vi "PH_Cont-601k_PSU.ProcCases.vi"(0 "i ref in":refnum<vi>, 1 "selector":string, 2 "Data":T1, 3 "call cluster":T2={"Object"="", "Selector"="", "CallType"=enum."synchronous", "Async Object"="", "Async Selector"="", "Data Descriptor"="", "Data"=[], "Error #"=0, "Expire"=0}, 5 "error in (no error)":errorcluster) -> (14 "i ref out":refnum<vi>, 17 "answer cluster":T2={"Object"="", "Selector"="", "CallType"=enum."synchronous", "Async Object"="", "Async Selector"="", "Data Descriptor"="", "Data"=[], "Error #"=0, "Expire"=0}, 19 "error out":errorcluster)   [LabVIEW 2014, in "PH_Cont-601k_PSU.lvlib"]
doc: "This method is called by a process from within the default case in the event loop. The methods of a class that are linked to events will be called from THIS method. Add your code here."
uses:
  PH_Cont-601k_PSU.lvlib
  CS_Core/CSSystem/CoreDefs/CoreDefs.call_type.ctl
  CS_Core/BaseProcess/BaseProcess.descriptor string definition.ctl
  CS_Core/CSSystem/CoreDefs/CoreDefs.rawDataType.ctl
  PH_Cont-601k_PSU.Readyness Device.ctl
  PH_Cont-601k_PSU.Readyness Program.ctl
  CS_Core/CSSystem/CoreLib/CoreLib.string 2 byte array.vi
  CS_Core/CSSystem/CoreLib/CoreLib.byte array 2 int.vi
  CS_Core/CSSystem/CoreLib/CoreLib.byte array 2 short.vi
  CS_Core/CSSystem/CoreLib/CoreLib.byte array 2 double.vi
  CS_Core/BaseProcess/BaseProcess.lvlib
  CS_Core/CSSystem/CoreLib/CoreLib.lvlib
  CS_Core/CAEObj/CAEObj.lvlib
  PH_Basics/PH_Common/PH_Common.lvlib
  PH_Basics/PH_Class/PH_Class.lvlib
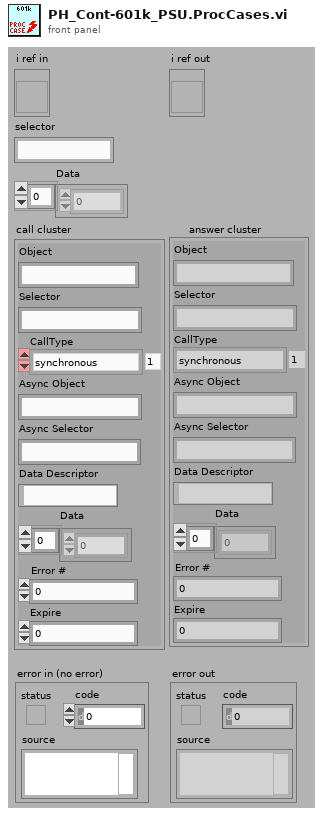
[diagram p1: front panel]
types:
  T1 = typedef "CoreDefs.rawDataType.ctl" = i8[]
  T2 = typedef "CoreDefs.call_type.ctl" = cluster{"Object":string, "Selector":string, "CallType":enum16{"simple", "synchronous", "asynchronous"}, "Async Object":string, "Async Selector":string, "Data Descriptor":T3, "Data":T1, "Error #":i32, "Expire":u32}
  T3 = typedef "BaseProcess.lvlib/BaseProcess.descriptor string definition.ctl" = string
  T4 = typedef "PH_Cont-601k_PSU.lvlib/PH_Cont-601k_PSU.Readyness Device.ctl" = enum32{"OFF", "CONNECTING", "CONNECTED", "OPERATING", "EOC", "ERROR"}
  T5 = typedef "PH_Cont-601k_PSU.lvlib/PH_Cont-601k_PSU.Readyness Program.ctl" = enum32{"OFF", "POWER", "INTERLOCK"}
  T6 = typedef "PH_Cont-601k_PSU.lvlib/PH_Cont-601k_PSU.Mode.ctl" = enum32{"STOP", "STANDBY", "READY", "EMISSION", "ERROR"}
  T7 = typedef "PH_Cont-601k_PSU.lvlib/PH_Cont-601k_PSU.i attribute.ctl" = cluster{"GUI Refs":T8, "Interlock":bool, "Service ID applied Voltage":i32, "Device Settings":cluster{"Configuration":T9, "Flash Interval [s]":dbl, "Mode":T6, "Voltage [V]":u16, "Charge":bool, "VISA resource name":refnum<visa-resource-name>}, "Readyness":T10, "Information":cluster{"VISA resource name":refnum<visa-resource-name>, "Tagname Power On":string, "Interlock":cluster{"Instance":string, "Tagname":string}, "Limits [V]":cluster{"Lower":dbl, "Upper":dbl}, "Tagname PSU On":string}, "R2S":bool, "Charge is allowed":bool}
  T8 = typedef "PH_Cont-601k_PSU.lvlib/PH_Cont-601k_PSU.GUI Refs.ctl" = cluster{"Power On":refnum<vi>, "Hard- and Software":refnum<vi>, "Device Status":refnum<vi>, "Device Error":refnum<vi>, "Configuration":refnum<vi>, "Flash Interval [s]":refnum<vi>, "Interlock":refnum<vi>, "Interlock Indicator":refnum<vi>, "Voltage [V]":refnum<vi>, "Readyness":refnum<vi>, "Mode":refnum<vi>, "Reset Error":refnum<vi>, "Expert working":refnum<vi>, "Charge":refnum<vi>, "PSU On":refnum<vi>}
  T9 = typedef "PH_Cont-601k_PSU.lvlib/PH_Cont-601k_PSU.Configuration.ctl" = u16
  T10 = typedef "PH_Cont-601k_PSU.lvlib/PH_Cont-601k_PSU.Readyness.ctl" = cluster{"Program":T5, "Device":T4}
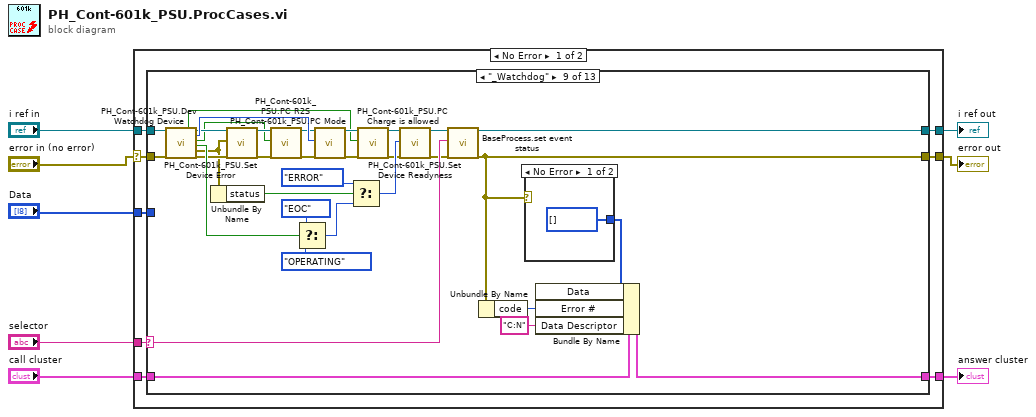
[diagram p0: block diagram]
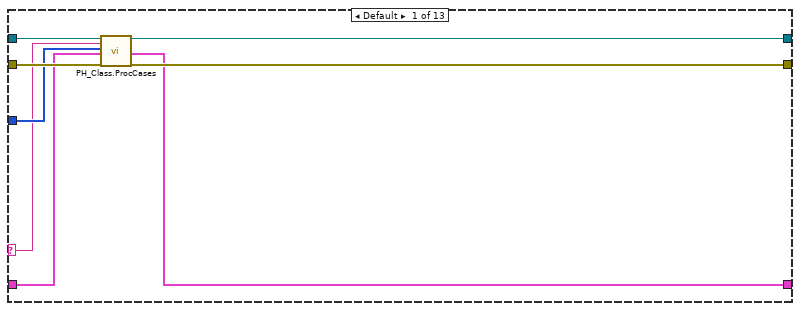
[diagram p2: hidden frame]
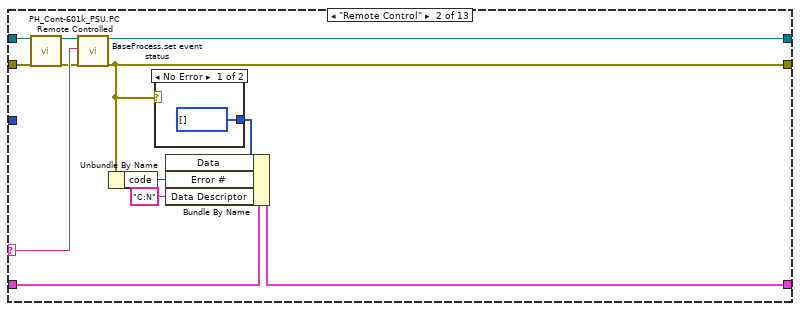
[diagram p3: hidden frame]
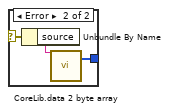
[diagram p4: hidden frame]
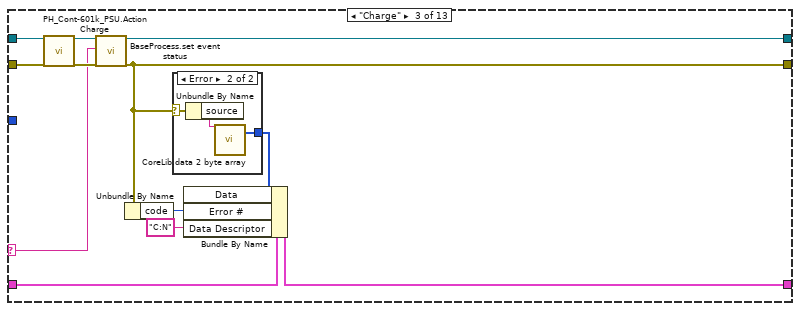
[diagram p5: hidden frame]
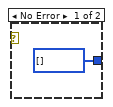
[diagram p6: hidden frame]
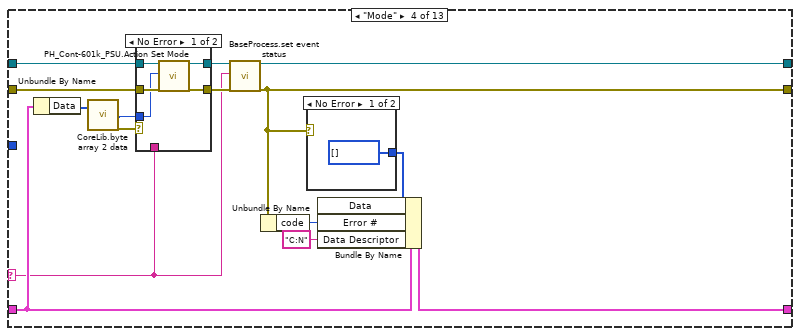
[diagram p7: hidden frame]
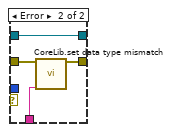
[diagram p8: hidden frame]
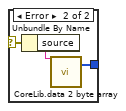
[diagram p9: hidden frame]
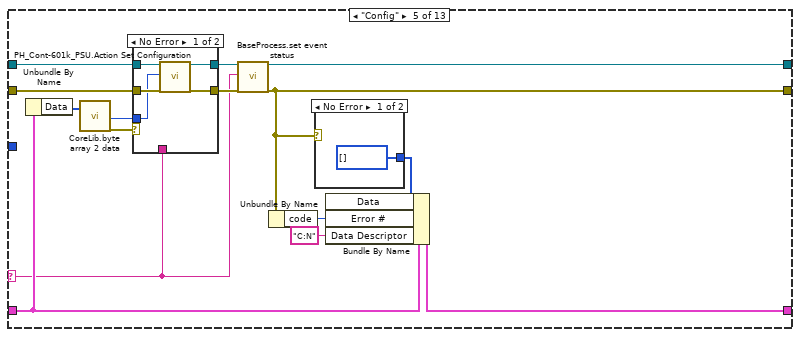
[diagram p10: hidden frame]
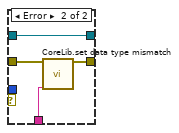
[diagram p11: hidden frame]
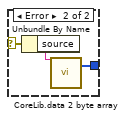
[diagram p12: hidden frame]
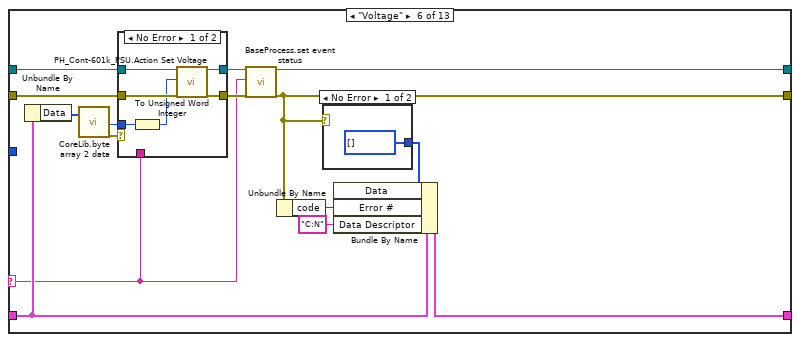
[diagram p13: hidden frame]
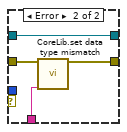
[diagram p14: hidden frame]
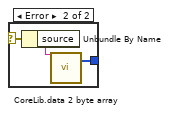
[diagram p15: hidden frame]
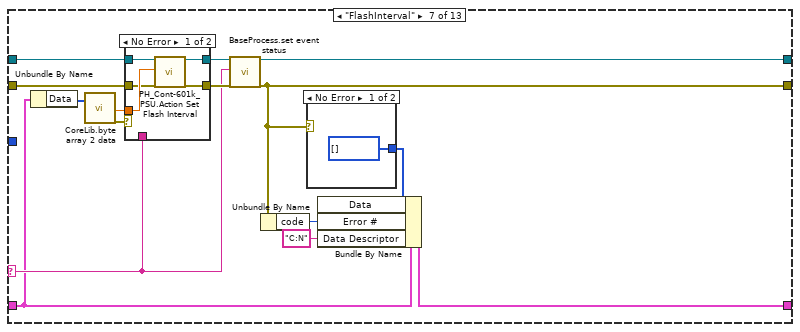
[diagram p16: hidden frame]
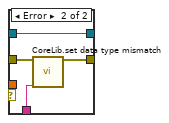
[diagram p17: hidden frame]
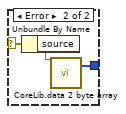
[diagram p18: hidden frame]
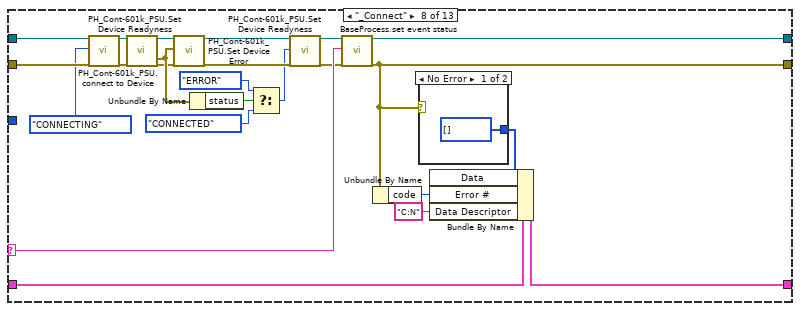
[diagram p19: hidden frame]
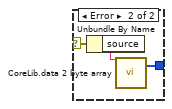
[diagram p20: hidden frame]
diagram:
  n1 = case shown="No Error" "error in (no error)" {
    selector: "error in (no error)" -> [w9 w425]
    tunnel: "selector" -> [w16 _]
    tunnel: [w15 w426] -> w7
    tunnel: "Data" -> [w14 _]
    tunnel: "call cluster" -> [w13 w426]
    tunnel: "i ref in" -> [w12 w427]
    tunnel: [w11 w427] -> w3
    tunnel: [w10 w425] -> w2
    frame No Error {
      n2 = case shown="\"_Watchdog\"" w16 {
        selector: w16 -> [w18 w32 w42 w57 w85 w113 w148 w186 w223 w240 w271 w319 w369]
        tunnel: w14 -> [w19 _ _ _ _ _ _ _ _ _ w270 w318 w368]
        tunnel: w12 -> [w17 w35 w41 w63 w91 w119 w147 w176 w211 w236 w264 w312 w362]
        tunnel: [w24 w27 w49 w68 w96 w124 w153 w190 w227 w246 w277 w325 w375] -> w11
        tunnel: w13 -> [w20 w30 w43 w60 w88 w116 w144 w187 w224 w241 w274 w322 w372]
        tunnel: [w21 w29 w50 w69 w97 w125 w154 w191 w228 w247 w280 w328 w378] -> w15
        tunnel: w9 -> [w23 w36 w46 w62 w90 w118 w146 w174 w210 w235 w275 w323 w373]
        tunnel: [w22 w26 w48 w67 w95 w123 w152 w189 w226 w245 w278 w326 w376] -> w10
        frame Default {
          n3 = call "PH_Class.ProcCases.vi"("i ref in"=w17, "selector"=w18, "Data"=w19, "call cluster"=w20, "error in (no error)"=w23) -> ("i ref out"=w24:refnum<vi>, "answer cluster"=w21:T2, "error out"=w22:errorcluster)  [unwired: 12 in]
        }
        frame "Remote Control" {
          n4 = call "PH_Cont-601k_PSU.PC Remote Controlled.vi"("i ref in"=w35, "error in (no error)"=w36) -> ("i ref out"=w31:refnum<vi>, "error out"=w28:errorcluster)  [unwired: 16 in]
          n5 = call "BaseProcess.set event status.vi"("i ref in"=w31, "EventStatus"=w32, "error in (no error)"=w28) -> ("i ref out"=w27:refnum<vi>, "error out"=w26:errorcluster)  [unwired: 14 in, 1 out]
          n6 = Unbundle By Name(w26) -> ("code"=w34:i32)
          n7 = case shown="No Error" w26 {
            selector: w26 -> [_ w40]
            tunnel: [T1 [] ("byteArray out") w39] -> w33
            frame No Error {
            }
            frame Error {
              n8 = Unbundle By Name(w40) -> ("source"=w38:string)
              n9 = call-poly "CoreLib.data 2 byte array.vi"("string"=w38) -> ("byteArray out"=w39:T1)  [unwired: 18 in]
            }
          }
          n10 = Bundle By Name(cluster=w30, "Data"=w33, "Error #"=w34, "Data Descriptor"="C:N") -> (w29:T2)
        }
        frame "Charge" {
          n11 = call "PH_Cont-601k_PSU.Action Charge.vi"("VI in"=w41, "error in (no error)"=w46) -> ("VI out"=w45:refnum<vi>, "error out"=w44:errorcluster)  [unwired: 16 in]
          n12 = call "BaseProcess.set event status.vi"("i ref in"=w45, "EventStatus"=w42, "error in (no error)"=w44) -> ("i ref out"=w49:refnum<vi>, "error out"=w48:errorcluster)  [unwired: 14 in, 1 out]
          n13 = Unbundle By Name(w48) -> ("code"=w52:i32)
          n14 = case shown="Error" w48 {
            selector: w48 -> [_ w56]
            tunnel: [T1 [] ("byteArray out") w55] -> w51
            frame No Error {
            }
            frame Error {
              n15 = Unbundle By Name(w56) -> ("source"=w54:string)
              n16 = call-poly "CoreLib.data 2 byte array.vi"("string"=w54) -> ("byteArray out"=w55:T1)  [unwired: 18 in]
            }
          }
          n17 = Bundle By Name(cluster=w43, "Data"=w51, "Error #"=w52, "Data Descriptor"="C:N") -> (w50:T2)
        }
        frame "Mode" {
          n18 = Unbundle By Name(w60) -> ("Data"=w61:T1)
          n19 = call-poly "CoreLib.byte array 2 data.vi"("byteArray"=w61) -> ("i32"=w59:i32, "error out"=w58:errorcluster)  [unwired: 16 in, 1 out]
          n20 = case shown="No Error" w58 {
            tunnel: [w76 w78] -> w65
            tunnel: [w75 w77] -> w64
            tunnel: w63 -> [w74 w77]
            tunnel: w62 -> [w73 w80]
            tunnel: w59 -> [w72 _]
            tunnel: w57 -> [_ w79]
            frame No Error {
              n21 = call "PH_Cont-601k_PSU.Action Set Mode.vi"("VI in"=w74, "Mode"=w72, "error in (no error)"=w73) -> ("VI out"=w75:refnum<vi>, "error out"=w76:errorcluster)  [unwired: 15 in]
            }
            frame Error {
              n22 = call "CoreLib.set data type mismatch.vi"("error in (no error)"=w80, "error source"=w79) -> ("error out"=w78:errorcluster)  [unwired: 17 in]
            }
          }
          n23 = call "BaseProcess.set event status.vi"("i ref in"=w64, "EventStatus"=w57, "error in (no error)"=w65) -> ("i ref out"=w68:refnum<vi>, "error out"=w67:errorcluster)  [unwired: 14 in, 1 out]
          n24 = Unbundle By Name(w67) -> ("code"=w71:i32)
          n25 = case shown="No Error" w67 {
            selector: w67 -> [_ w84]
            tunnel: [T1 [] ("byteArray out") w83] -> w70
            frame No Error {
            }
            frame Error {
              n26 = Unbundle By Name(w84) -> ("source"=w82:string)
              n27 = call-poly "CoreLib.data 2 byte array.vi"("string"=w82) -> ("byteArray out"=w83:T1)  [unwired: 18 in]
            }
          }
          n28 = Bundle By Name(cluster=w60, "Data"=w70, "Error #"=w71, "Data Descriptor"="C:N") -> (w69:T2)
        }
        frame "Config" {
          n29 = Unbundle By Name(w88) -> ("Data"=w89:T1)
          n30 = call-poly "CoreLib.byte array 2 data.vi"("byteArray"=w89) -> ("i16"=w87:i16, "error out"=w86:errorcluster)  [unwired: 16 in, 1 out]
          n31 = case shown="No Error" w86 {
            tunnel: [w104 w107] -> w93
            tunnel: [w103 w106] -> w92
            tunnel: w91 -> [w102 w106]
            tunnel: w90 -> [w101 w108]
            tunnel: w87 -> [w100 _]
            tunnel: w85 -> [_ w105]
            frame No Error {
              n32 = call "PH_Cont-601k_PSU.Action Set Configuration.vi"("VI in"=w102, "Configuration"=w100, "error in (no error)"=w101) -> ("VI out"=w103:refnum<vi>, "error out"=w104:errorcluster)  [unwired: 15 in]
            }
            frame Error {
              n33 = call "CoreLib.set data type mismatch.vi"("error in (no error)"=w108, "error source"=w105) -> ("error out"=w107:errorcluster)  [unwired: 17 in]
            }
          }
          n34 = call "BaseProcess.set event status.vi"("i ref in"=w92, "EventStatus"=w85, "error in (no error)"=w93) -> ("i ref out"=w96:refnum<vi>, "error out"=w95:errorcluster)  [unwired: 14 in, 1 out]
          n35 = Unbundle By Name(w95) -> ("code"=w99:i32)
          n36 = case shown="No Error" w95 {
            selector: w95 -> [_ w112]
            tunnel: [T1 [] ("byteArray out") w111] -> w98
            frame No Error {
            }
            frame Error {
              n37 = Unbundle By Name(w112) -> ("source"=w110:string)
              n38 = call-poly "CoreLib.data 2 byte array.vi"("string"=w110) -> ("byteArray out"=w111:T1)  [unwired: 18 in]
            }
          }
          n39 = Bundle By Name(cluster=w88, "Data"=w98, "Error #"=w99, "Data Descriptor"="C:N") -> (w97:T2)
        }
        frame "Voltage" {
          n40 = Unbundle By Name(w116) -> ("Data"=w117:T1)
          n41 = call-poly "CoreLib.byte array 2 data.vi"("byteArray"=w117) -> ("i16"=w114:i16, "error out"=w115:errorcluster)  [unwired: 16 in, 1 out]
          n42 = case shown="No Error" w115 {
            tunnel: [w133 w136] -> w121
            tunnel: [w132 w134] -> w120
            tunnel: w119 -> [w131 w134]
            tunnel: w118 -> [w130 w137]
            tunnel: w114 -> [w129 _]
            tunnel: w113 -> [_ w135]
            frame No Error {
              n43 = To Unsigned Word Integer(number=w129) -> (unsigned 16bit integer=w128:u16)
              n44 = call "PH_Cont-601k_PSU.Action Set Voltage.vi"("VI in"=w131, "Voltage [V]"=w128, "error in (no error)"=w130) -> ("VI out"=w132:refnum<vi>, "error out"=w133:errorcluster)  [unwired: 15 in]
            }
            frame Error {
              n45 = call "CoreLib.set data type mismatch.vi"("error in (no error)"=w137, "error source"=w135) -> ("error out"=w136:errorcluster)  [unwired: 17 in]
            }
          }
          n46 = call "BaseProcess.set event status.vi"("i ref in"=w120, "EventStatus"=w113, "error in (no error)"=w121) -> ("i ref out"=w124:refnum<vi>, "error out"=w123:errorcluster)  [unwired: 14 in, 1 out]
          n47 = Unbundle By Name(w123) -> ("code"=w127:i32)
          n48 = case shown="No Error" w123 {
            selector: w123 -> [_ w141]
            tunnel: [T1 [] ("byteArray out") w140] -> w126
            frame No Error {
            }
            frame Error {
              n49 = Unbundle By Name(w141) -> ("source"=w139:string)
              n50 = call-poly "CoreLib.data 2 byte array.vi"("string"=w139) -> ("byteArray out"=w140:T1)  [unwired: 18 in]
            }
          }
          n51 = Bundle By Name(cluster=w116, "Data"=w126, "Error #"=w127, "Data Descriptor"="C:N") -> (w125:T2)
        }
        frame "FlashInterval" {
          n52 = Unbundle By Name(w144) -> ("Data"=w145:T1)
          n53 = call-poly "CoreLib.byte array 2 data.vi"("byteArray"=w145) -> ("d64"=w143:dbl, "error out"=w142:errorcluster)  [unwired: 16 in, 1 out]
          n54 = case shown="No Error" w142 {
            tunnel: [w161 w163] -> w150
            tunnel: [w160 w164] -> w149
            tunnel: w148 -> [_ w162]
            tunnel: w147 -> [w157 w164]
            tunnel: w146 -> [w158 w165]
            tunnel: w143 -> [w159 _]
            frame No Error {
              n55 = call "PH_Cont-601k_PSU.Action Set Flash Interval.vi"("VI in"=w157, "Flash Interval [s]"=w159, "error in (no error)"=w158) -> ("VI out"=w160:refnum<vi>, "error out"=w161:errorcluster)  [unwired: 15 in]
            }
            frame Error {
              n56 = call "CoreLib.set data type mismatch.vi"("error in (no error)"=w165, "error source"=w162) -> ("error out"=w163:errorcluster)  [unwired: 17 in]
            }
          }
          n57 = call "BaseProcess.set event status.vi"("i ref in"=w149, "EventStatus"=w148, "error in (no error)"=w150) -> ("i ref out"=w153:refnum<vi>, "error out"=w152:errorcluster)  [unwired: 14 in, 1 out]
          n58 = Unbundle By Name(w152) -> ("code"=w156:i32)
          n59 = case shown="No Error" w152 {
            selector: w152 -> [_ w169]
            tunnel: [T1 [] ("byteArray out") w168] -> w155
            frame No Error {
            }
            frame Error {
              n60 = Unbundle By Name(w169) -> ("source"=w167:string)
              n61 = call-poly "CoreLib.data 2 byte array.vi"("string"=w167) -> ("byteArray out"=w168:T1)  [unwired: 18 in]
            }
          }
          n62 = Bundle By Name(cluster=w144, "Data"=w155, "Error #"=w156, "Data Descriptor"="C:N") -> (w154:T2)
        }
        frame "_Connect" {
          n63 = call "PH_Cont-601k_PSU.Set Device Readyness.vi"("VI in"=w176, "Readyness Device to set"=PH_Cont-601k_PSU.Readyness_Device."CONNECTING", "error in (no error)"=w174) -> ("VI out"=w175:refnum<vi>, "error out"=w173:errorcluster)  [unwired: 15 in]
          n64 = call "PH_Cont-601k_PSU.connect to Device.vi"("VI in"=w175, "error in (no error)"=w173) -> ("VI out"=w177:refnum<vi>, "Device Error out"=w179:errorcluster, "error out"=w178:errorcluster)  [unwired: 15 in]
          n65 = call "PH_Cont-601k_PSU.Set Device Error.vi"("VI in"=w177, "Device Error"=w179, "error in (no error)"=w178) -> ("VI out"=w184:refnum<vi>, "error out"=w185:errorcluster)  [unwired: 15 in]
          n66 = Unbundle By Name(w179) -> ("status"=w181:bool)
          n67 = Select(t=PH_Cont-601k_PSU.Readyness_Device."ERROR" ("Readyness.Device"), s=w181, f=PH_Cont-601k_PSU.Readyness_Device."CONNECTED" ("Readyness Device to set")) -> (s? t:f=w183:T4)
          n68 = call "PH_Cont-601k_PSU.Set Device Readyness.vi"("VI in"=w184, "Readyness Device to set"=w183, "error in (no error)"=w185) -> ("VI out"=w171:refnum<vi>, "error out"=w170:errorcluster)  [unwired: 15 in]
          n69 = call "BaseProcess.set event status.vi"("i ref in"=w171, "EventStatus"=w186, "error in (no error)"=w170) -> ("i ref out"=w190:refnum<vi>, "error out"=w189:errorcluster)  [unwired: 14 in, 1 out]
          n70 = Unbundle By Name(w189) -> ("code"=w193:i32)
          n71 = case shown="No Error" w189 {
            selector: w189 -> [_ w197]
            tunnel: [T1 [] ("byteArray out") w196] -> w192
            frame No Error {
            }
            frame Error {
              n72 = Unbundle By Name(w197) -> ("source"=w195:string)
              n73 = call-poly "CoreLib.data 2 byte array.vi"("string"=w195) -> ("byteArray out"=w196:T1)  [unwired: 18 in]
            }
          }
          n74 = Bundle By Name(cluster=w187, "Data"=w192, "Error #"=w193, "Data Descriptor"="C:N") -> (w191:T2)
        }
        frame "_Watchdog" {
          n75 = call "PH_Cont-601k_PSU.Dev Watchdog Device.vi"("VI in"=w211, "error in (no error)"=w210) -> ("Charge is allowed"=w198:bool, "VI out"=w215:refnum<vi>, "Mode"=w216:T6, "R2S"=w203:bool, "EOC reached?"=w221:bool, "Device Error out"=w212:errorcluster, "error out"=w214:errorcluster)  [unwired: 11 in]
          n76 = Unbundle By Name(w212) -> ("status"=w213:bool)
          n77 = call "PH_Cont-601k_PSU.Set Device Error.vi"("VI in"=w215, "Device Error"=w212, "error in (no error)"=w214) -> ("VI out"=w207:refnum<vi>, "error out"=w206:errorcluster)  [unwired: 15 in]
          n78 = call "PH_Cont-601k_PSU.PC R2S.vi"("VI in"=w207, "R2S"=w203, "error in (no error)"=w206) -> ("VI out"=w205:refnum<vi>, "error out"=w204:errorcluster)  [unwired: 14 in, 1 out]
          n79 = Select(t=PH_Cont-601k_PSU.Readyness_Device."EOC" ("Readyness.Device"), s=w221, f=PH_Cont-601k_PSU.Readyness_Device."OPERATING" ("Readyness.Device")) -> (s? t:f=w220:T4)
          n80 = call "PH_Cont-601k_PSU.PC Mode.vi"("VI in"=w205, "Mode"=w216, "error in (no error)"=w204) -> ("VI out"=w200:refnum<vi>, "error out"=w202:errorcluster)  [unwired: 14 in, 1 out]
          n81 = Select(t=PH_Cont-601k_PSU.Readyness_Device."ERROR" ("Readyness.Device"), s=w213, f=w220) -> (s? t:f=w217:T4)
          n82 = call "PH_Cont-601k_PSU.PC Charge is allowed.vi"("VI in"=w200, "Charge is allowed"=w198, "error in (no error)"=w202) -> ("VI out"=w199:refnum<vi>, "error out"=w201:errorcluster)  [unwired: 14 in, 1 out]
          n83 = call "PH_Cont-601k_PSU.Set Device Readyness.vi"("VI in"=w199, "Readyness Device to set"=w217, "error in (no error)"=w201) -> ("VI out"=w209:refnum<vi>, "error out"=w208:errorcluster)  [unwired: 15 in]
          n84 = call "BaseProcess.set event status.vi"("i ref in"=w209, "EventStatus"=w223, "error in (no error)"=w208) -> ("i ref out"=w227:refnum<vi>, "error out"=w226:errorcluster)  [unwired: 14 in, 1 out]
          n85 = Unbundle By Name(w226) -> ("code"=w230:i32)
          n86 = case shown="No Error" w226 {
            selector: w226 -> [_ w234]
            tunnel: [T1 [] ("byteArray out") w233] -> w229
            frame No Error {
            }
            frame Error {
              n87 = Unbundle By Name(w234) -> ("source"=w232:string)
              n88 = call-poly "CoreLib.data 2 byte array.vi"("string"=w232) -> ("byteArray out"=w233:T1)  [unwired: 18 in]
            }
          }
          n89 = Bundle By Name(cluster=w224, "Data"=w229, "Error #"=w230, "Data Descriptor"="C:N") -> (w228:T2)
        }
        frame "Interlock" {
          n90 = Unbundle By Name(w241) -> ("Data"=w239:T1)
          n91 = call-poly "CoreLib.byte array 2 data.vi"("byteArray"=w239) -> ("i16"=w237:i16, "error out"=w238:errorcluster)  [unwired: 16 in, 1 out]
          n92 = case shown="No Error" w238 {
            tunnel: w235 -> [w251 w258]
            tunnel: [w253 w257] -> w243
            tunnel: w236 -> [w252 w259]
            tunnel: [w254 w259] -> w242
            tunnel: w237 -> [w255 _]
            tunnel: w240 -> [_ w256]
            frame No Error {
              n93 = Greater Than 0?(x=w255) -> (x > 0?=w250:bool)
              n94 = call "PH_Cont-601k_PSU.PC Set Interlock.vi"("VI in"=w252, "Set Interlock"=w250, "error in (no error)"=w251) -> ("VI out"=w254:refnum<vi>, "error out"=w253:errorcluster)  [unwired: 15 in]
            }
            frame Error {
              n95 = call "CoreLib.set data type mismatch.vi"("error in (no error)"=w258, "error source"=w256) -> ("error out"=w257:errorcluster)  [unwired: 17 in]
            }
          }
          n96 = call "BaseProcess.set event status.vi"("i ref in"=w242, "EventStatus"=w240, "error in (no error)"=w243) -> ("i ref out"=w246:refnum<vi>, "error out"=w245:errorcluster)  [unwired: 14 in, 1 out]
          n97 = Unbundle By Name(w245) -> ("code"=w249:i32)
          n98 = case shown="No Error" w245 {
            selector: w245 -> [_ w263]
            tunnel: [T1 [] ("byteArray out") w262] -> w248
            frame No Error {
            }
            frame Error {
              n99 = Unbundle By Name(w263) -> ("source"=w261:string)
              n100 = call-poly "CoreLib.data 2 byte array.vi"("string"=w261) -> ("byteArray out"=w262:T1)  [unwired: 18 in]
            }
          }
          n101 = Bundle By Name(cluster=w241, "Data"=w248, "Error #"=w249, "Data Descriptor"="C:N") -> (w247:T2)
        }
        frame "_Power On" {
          n102 = call "CAEObj.unfold trend data.vi"("i ref in"=w264, "raw trend data"=w270) -> ("quality"=w268:i32, "no link"=w266:bool, "data"=w267:i8[], "typeDescriptor"=w265:string, "error out"=w269:errorcluster)  [unwired: 9 in, 4 out]
          n103 = case shown="No Error" w269 {
            tunnel: [w285 w307] -> w273
            tunnel: w264 -> [w303 w307]
            tunnel: w275 -> [w302 w306]
            tunnel: [w283 w305] -> w272
            tunnel: w271 -> [_ w304]
            tunnel: w268 -> [w299 _]
            tunnel: w267 -> [w298 _]
            tunnel: w266 -> [w295 _]
            tunnel: w265 -> [w297 _]
            frame No Error {
              n104 = call "PH_Cont-601k_PSU.get i attribute.vi"("i ref in"=w303, "error in (no error)"=w302) -> ("i ref out"=w289:refnum<vi>, "i attribute"=w300:T7, "error out"=w301:errorcluster)  [unwired: 15 in]
              n105 = call "PH_DIM.get Boolean.vi"("no link"=w295, "typeDescriptor"=w297, "data"=w298, "quality"=w299) -> ("Value"=w296:i32)
              n106 = Unbundle By Name(w300) -> ("GUI Refs.Power On"=w294:refnum<vi>)
              n107 = Equal?(x=w296, y=2) -> (x = y?=w292:bool)
              n108 = call "PH_GUI.set color GUI object.vi"("GUI object Ref"=w294, "State"=w296, "Blinking? (false)"=w295, "error in (no error)"=w301) -> ("error out"=w288:errorcluster)  [unwired: 15 in]
              n109 = Select(t=PH_Cont-601k_PSU.Readyness_Program."POWER" ("Readyness.Program"), s=w292, f=PH_Cont-601k_PSU.Readyness_Program."OFF") -> (s? t:f=w287:T5)
              n110 = call "PH_Cont-601k_PSU.Set Readyness - Program.vi"("VI in"=w289, "Readyness - Program"=w287, "error in (no error)"=w288) -> ("VI out"=w286:refnum<vi>, "error out"=w284:errorcluster)  [unwired: 15 in]
              n111 = call "PH_Cont-601k_PSU.PC Set Interlock.vi"("VI in"=w286, "Set Interlock"=FALSE, "error in (no error)"=w284) -> ("VI out"=w285:refnum<vi>, "error out"=w283:errorcluster)  [unwired: 15 in]
            }
            frame Error {
              n112 = call "CoreLib.set data type mismatch.vi"("error in (no error)"=w306, "error source"=w304) -> ("error out"=w305:errorcluster)  [unwired: 17 in]
            }
          }
          n113 = call "BaseProcess.set event status.vi"("i ref in"=w273, "EventStatus"=w271, "error in (no error)"=w272) -> ("i ref out"=w277:refnum<vi>, "error out"=w278:errorcluster)  [unwired: 14 in, 1 out]
          n114 = Unbundle By Name(w278) -> ("code"=w281:i32)
          n115 = case shown="No Error" w278 {
            selector: w278 -> [_ w311]
            tunnel: [T1 [] ("byteArray out") w310] -> w279
            frame No Error {
            }
            frame Error {
              n116 = Unbundle By Name(w311) -> ("source"=w309:string)
              n117 = call-poly "CoreLib.data 2 byte array.vi"("string"=w309) -> ("byteArray out"=w310:T1)  [unwired: 18 in]
            }
          }
          n118 = Bundle By Name(cluster=w274, "Data"=w279, "Error #"=w281, "Data Descriptor"="C:N") -> (w280:T2)
        }
        frame "_PSU On" {
          n119 = call "CAEObj.unfold trend data.vi"("i ref in"=w312, "raw trend data"=w318) -> ("quality"=w316:i32, "no link"=w314:bool, "data"=w315:i8[], "typeDescriptor"=w313:string, "error out"=w317:errorcluster)  [unwired: 9 in, 4 out]
          n120 = case shown="No Error" w317 {
            tunnel: [w334 w357] -> w321
            tunnel: w312 -> [w343 w357]
            tunnel: w323 -> [w342 w356]
            tunnel: [w333 w355] -> w320
            tunnel: w319 -> [_ w354]
            tunnel: w316 -> [w339 _]
            tunnel: w315 -> [w338 _]
            tunnel: w314 -> [w336 _]
            tunnel: w313 -> [w337 _]
            frame No Error {
              n121 = call "PH_Cont-601k_PSU.get i attribute.vi"("i ref in"=w343, "error in (no error)"=w342) -> ("i ref out"=w334:refnum<vi>, "i attribute"=w340:T7, "error out"=w341:errorcluster)  [unwired: 15 in]
              n122 = call "PH_DIM.get Boolean.vi"("no link"=w336, "typeDescriptor"=w337, "data"=w338, "quality"=w339) -> ("Value"=w331:i32)
              n123 = Unbundle By Name(w340) -> ("GUI Refs.PSU On"=w335:refnum<vi>, "Readyness.Program"=w332:T5)
              n124 = case shown="Default" w332 {
                tunnel: w331 -> [w346 w351]
                tunnel: [w345 w350] -> w330
                frame "OFF" {
                  n125 = Equal?(x=2, y=w346) -> (x = y?=w347:bool)
                  n126 = Select(t=3, s=w347, f=w346) -> (s? t:f=w345:i32)
                }
                frame Default {
                  n127 = Equal?(x=1, y=w351) -> (x = y?=w352:bool)
                  n128 = Select(t=3, s=w352, f=w351) -> (s? t:f=w350:i32)
                }
              }
              n129 = call "PH_GUI.set color GUI object.vi"("GUI object Ref"=w335, "State"=w330, "Blinking? (false)"=w336, "error in (no error)"=w341) -> ("error out"=w333:errorcluster)  [unwired: 15 in]
            }
            frame Error {
              n130 = call "CoreLib.set data type mismatch.vi"("error in (no error)"=w356, "error source"=w354) -> ("error out"=w355:errorcluster)  [unwired: 17 in]
            }
          }
          n131 = call "BaseProcess.set event status.vi"("i ref in"=w321, "EventStatus"=w319, "error in (no error)"=w320) -> ("i ref out"=w325:refnum<vi>, "error out"=w326:errorcluster)  [unwired: 14 in, 1 out]
          n132 = Unbundle By Name(w326) -> ("code"=w329:i32)
          n133 = case shown="No Error" w326 {
            selector: w326 -> [_ w361]
            tunnel: [T1 [] ("byteArray out") w360] -> w327
            frame No Error {
            }
            frame Error {
              n134 = Unbundle By Name(w361) -> ("source"=w359:string)
              n135 = call-poly "CoreLib.data 2 byte array.vi"("string"=w359) -> ("byteArray out"=w360:T1)  [unwired: 18 in]
            }
          }
          n136 = Bundle By Name(cluster=w322, "Data"=w327, "Error #"=w329, "Data Descriptor"="C:N") -> (w328:T2)
        }
        frame "_Interlock" {
          n137 = call "CAEObj.unfold trend data.vi"("i ref in"=w362, "raw trend data"=w368) -> ("quality"=w366:i32, "no link"=w364:bool, "data"=w365:i8[], "typeDescriptor"=w363:string, "error out"=w367:errorcluster)  [unwired: 9 in, 4 out]
          n138 = case shown="No Error" w367 {
            tunnel: [w393 w420] -> w371
            tunnel: w362 -> [w409 w420]
            tunnel: w373 -> [w408 w419]
            tunnel: [w395 w418] -> w370
            tunnel: w369 -> [_ w417]
            tunnel: w366 -> [w405 _]
            tunnel: w365 -> [w404 _]
            tunnel: w364 -> [w402 _]
            tunnel: w363 -> [w403 _]
            frame No Error {
              w384 = PH_Cont-601k_PSU.Readyness_Program."OFF" ("y")
              n139 = call "PH_Cont-601k_PSU.get i attribute.vi"("i ref in"=w409, "error in (no error)"=w408) -> ("i ref out"=w397:refnum<vi>, "i attribute"=w406:T7, "error out"=w407:errorcluster)  [unwired: 15 in]
              n140 = call "PH_DIM.get Boolean.vi"("no link"=w402, "typeDescriptor"=w403, "data"=w404, "quality"=w405) -> ("Value"=w389:i32)
              n141 = Unbundle By Name(w406) -> ("GUI Refs.Interlock"=w399:refnum<vi>, "GUI Refs.Interlock Indicator"=w400:refnum<vi>, "Readyness.Program"=w382:T5)
              n142 = Equal?(x=w389, y=0) -> (x = y?=w388:bool)
              n143 = Equal?(x=w389, y=2) -> (x = y?=w381:bool)
              n144 = Select(t=PH_Cont-601k_PSU.Readyness_Program."INTERLOCK" ("y"), s=w381, f=PH_Cont-601k_PSU.Readyness_Program."POWER") -> (s? t:f=w380:T5)
              n145 = Equal?(x=w384, y=w382) -> (x = y?=w391:bool)
              n146 = call "PH_GUI.set color GUI object.vi"("GUI object Ref"=w400, "State"=w389, "Blinking? (false)"=w402, "error in (no error)"=w407) -> ("error out"=w401:errorcluster)  [unwired: 15 in]
              n147 = Select(t=w384, s=w388, f=w380) -> (s? t:f=w387:T5)
              n148 = call "PH_GUI.set boolean GUI object.vi"("Boolean Knob GUI Ref"=w399, "Value"=w381, "error in (no error)"=w401) -> ("error out"=w398:errorcluster)  [unwired: 16 in]
              n149 = Select(t=w384, s=w391, f=w387) -> (s? t:f=w390:T5)
              n150 = call "PH_Cont-601k_PSU.Set Readyness - Program.vi"("VI in"=w397, "Readyness - Program"=w390, "error in (no error)"=w398) -> ("VI out"=w394:refnum<vi>, "error out"=w396:errorcluster)  [unwired: 15 in]
              n151 = case shown="Default" w390 {
                tunnel: w396 -> [w411 w416]
                tunnel: [w411 w415] -> w395
                tunnel: w394 -> [w410 w414]
                tunnel: [w410 w413] -> w393
                frame Default {
                }
                frame "OFF" {
                  n152 = call "PH_Cont-601k_PSU.PC Set Interlock.vi"("VI in"=w414, "Set Interlock"=FALSE, "error in (no error)"=w416) -> ("VI out"=w413:refnum<vi>, "error out"=w415:errorcluster)  [unwired: 15 in]
                }
              }
            }
            frame Error {
              n153 = call "CoreLib.set data type mismatch.vi"("error in (no error)"=w419, "error source"=w417) -> ("error out"=w418:errorcluster)  [unwired: 17 in]
            }
          }
          n154 = call "BaseProcess.set event status.vi"("i ref in"=w371, "EventStatus"=w369, "error in (no error)"=w370) -> ("i ref out"=w375:refnum<vi>, "error out"=w376:errorcluster)  [unwired: 14 in, 1 out]
          n155 = Unbundle By Name(w376) -> ("code"=w379:i32)
          n156 = case shown="No Error" w376 {
            selector: w376 -> [_ w424]
            tunnel: [T1 [] ("byteArray out") w423] -> w377
            frame No Error {
            }
            frame Error {
              n157 = Unbundle By Name(w424) -> ("source"=w422:string)
              n158 = call-poly "CoreLib.data 2 byte array.vi"("string"=w422) -> ("byteArray out"=w423:T1)  [unwired: 18 in]
            }
          }
          n159 = Bundle By Name(cluster=w372, "Data"=w377, "Error #"=w379, "Data Descriptor"="C:N") -> (w378:T2)
        }
      }
    }
    frame Error {
    }
  }
  "answer cluster" <- w7
  "i ref out" <- w3
  "error out" <- w2
